vi "EOL CAN_Get_Motor_Constant_Level (2).vi"(11 "NetworkObjHandle":u32) -> (0 "Constant Level":string, 2 "TxRx Data":string[][](array[string]), 3 "Response Good?":bool)   [LabVIEW 2012]
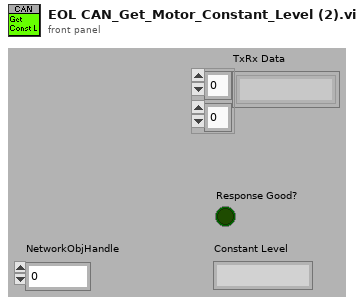
[diagram p1: front panel]
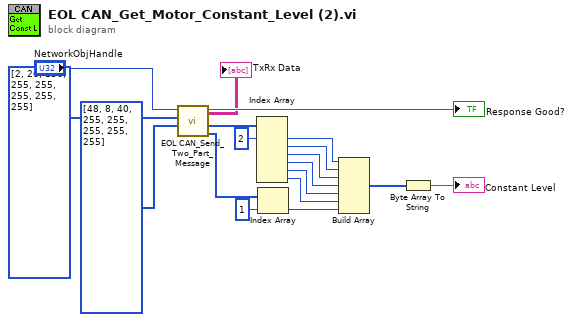
[diagram p0: block diagram]
diagram:
  n1 = call "EOL CAN_Send_Two_Part_Message.vi"("Tx 2"=u8[] [48, 8, 40, 255, 255, 255, 255, 255] ("Transmit Data"), "Tx 1"=u8[] [2, 26, 156, 255, 255, 255, 255, 255] ("Transmit Data"), "NetworkObjHandle"="NetworkObjHandle") -> ("Array 23"=w2:u8[], "Array 22"=w3:u8[], "Response Good?"=→"Response Good?":bool, "TxRx Data"=→"TxRx Data":string[][])  [unwired: 4 in, 1 out]
  n2 = Index Array(array=w3, index #1=2 ("index")) -> (element #1=w7:u8, element #2=w8:u8, element #3=w9:u8, element #4=w10:u8, element #5=w11:u8, element #6=w12:u8)  [unwired: 5 in]
  n3 = Index Array(array=w2, index=1) -> (element=w13:u8)
  n4 = Build Array(w7, w8, w9, w10, w11, w12, w13) -> (w14:u8[])
  n5 = Byte Array To String(unsigned byte array=w14) -> (string=→"Constant Level":string)
